vi "String to path.vi"(8 "error in (no error)":errorcluster, 11 "String":string) -> (0 "error out":errorcluster, 3 "appended path":path)   [LabVIEW 2023, in "User Sender.lvclass"]
uses:
  User Sender.lvclass
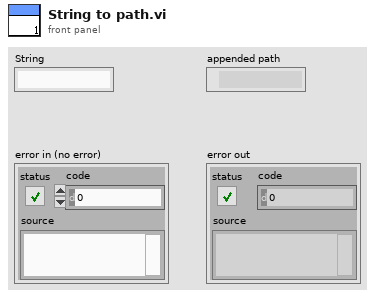
[diagram p1: front panel]
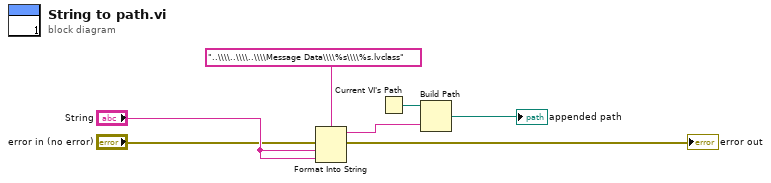
[diagram p0: block diagram]
diagram:
  n1 = Format Into String(format string="..\\\\..\\\\..\\\\Message Data\\\\%s\\\\%s.lvclass", error in="error in (no error)", "String", "String") -> (resulting string=w6:string, error out=→"error out":errorcluster)  [unwired: 1 in]
  n2 = Current VI's Path() -> (path=w7:path)
  n3 = Build Path(base path=w7, name or relative path=w6) -> (appended path=→"appended path":path)
